vi "Package Name.vi"(8 "error in (no error)":errorcluster, 11 "Build Specification Name":string) -> (0 "error out":errorcluster, 3 "Package Name":string)   [LabVIEW 2015]
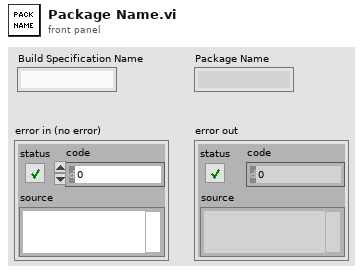
[diagram p1: front panel]
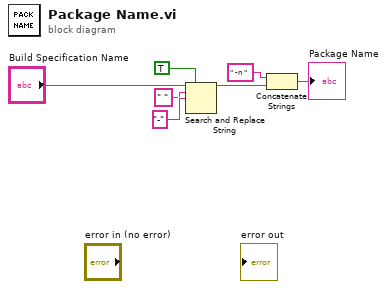
[diagram p0: block diagram]
diagram:
  n1 = Search and Replace String(replace all?=TRUE ("replace all? (F)"), input string="Build Specification Name", search string=" ", replace string="-" ("replace string (\"\")")) -> (result string=w2:string)  [unwired: 4 in, 3 out]
  n2 = Concatenate Strings(" -n " ("string"), w2) -> (→"Package Name":string)
